vi "Configure Limit Test.vi"(0 "VISA resource name":refnum<visa-resource-name>, 1 "Upper Fail Line (0)":i32, 2 "Lower Fail Line (0)":i32, 5 "Limit Number (0: Limit1)":i32(ring) items=["Limit1", "Limit2"], 7 "Enable Limit Test (F: Disable)":bool, 9 "Upper Limit (1.000000E+0)":dbl=1.0 format="%.6e", 11 "error in (no error)":errorcluster, 12 "Lower Limit (-1.000000E+0)":dbl=-1.0 format="%.6e", 13 "Auto Clear (T: Enable)":bool=TRUE) -> (4 "VISA resource name out":refnum<visa-resource-name>, 15 "error out":errorcluster)   [LabVIEW 2016, in "Keithley 6517.lvlib"]
doc: "Configures the LIMIT 1 or 2 for CALC 3(model 6517) or CALC2(model 6514) math calculation."
uses:
  <instrlib>/Keithley 6517/Keithley 6517.lvlib
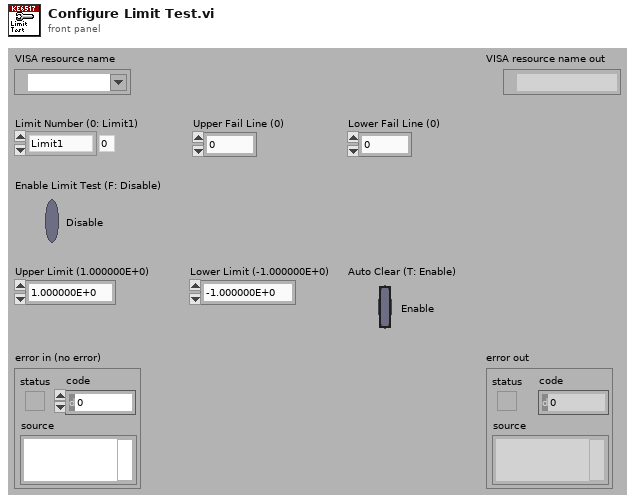
[diagram p1: front panel]
types:
  T1 = typedef "Keithley 6517.lvlib/Extended User Data.ctl" = cluster{"Instrument Model":i32}
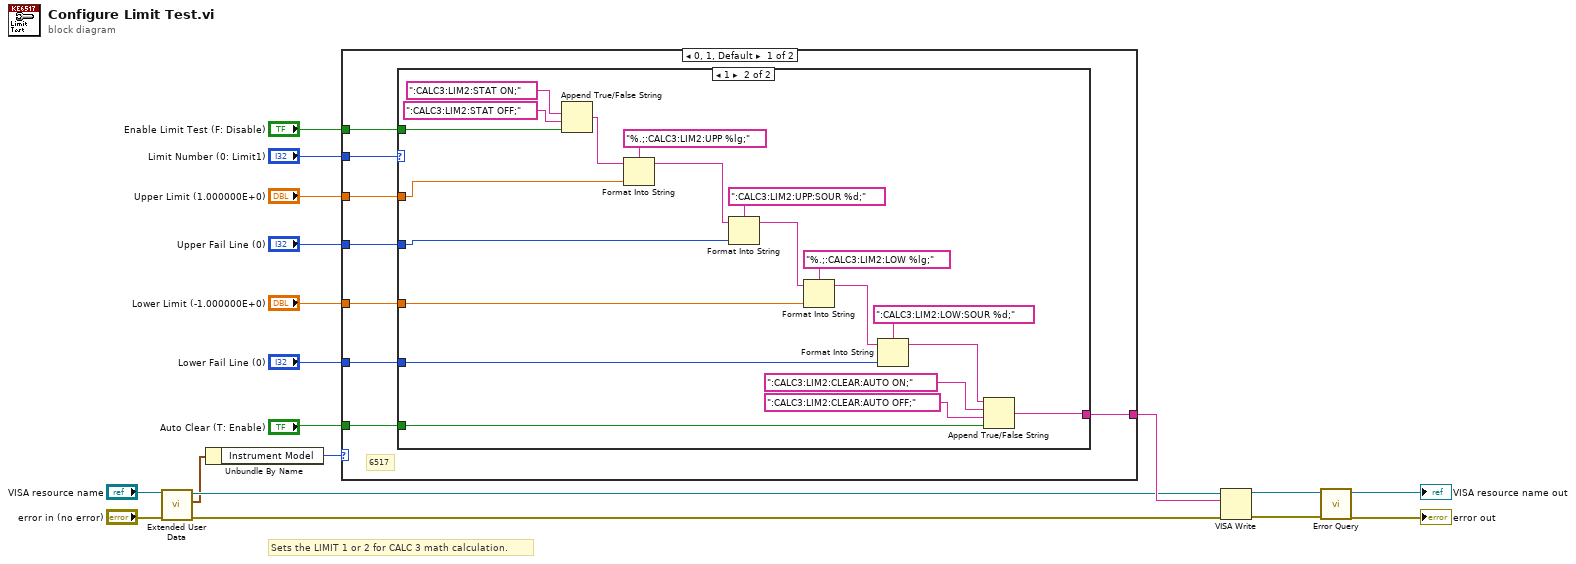
[diagram p0: block diagram]
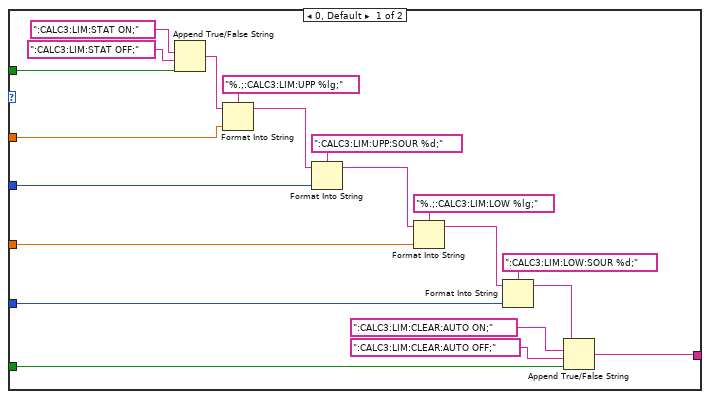
[diagram p2: hidden frame]
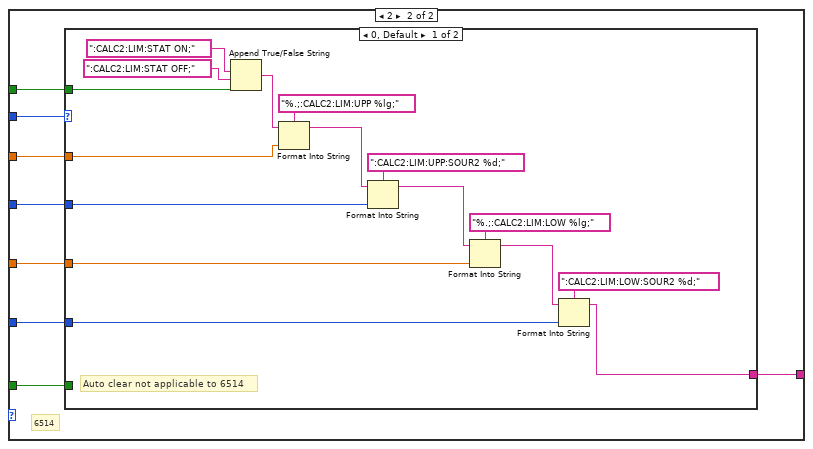
[diagram p3: hidden frame]
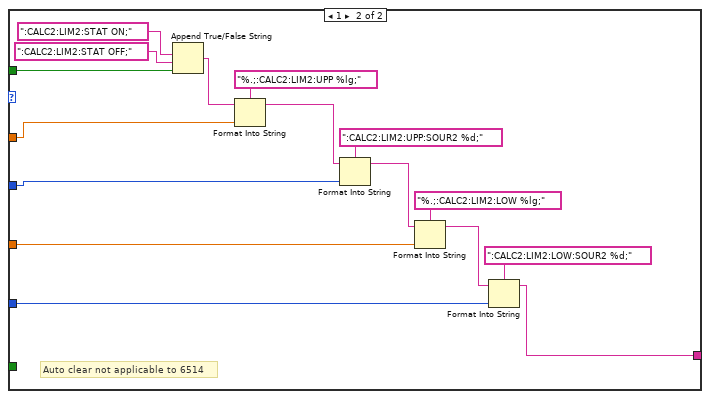
[diagram p4: hidden frame]
diagram:
  # "Sets the LIMIT 1 or 2 for CALC 3 math calculation."
  n1 = call <instrlib>:"Extended User Data.vi"("error in (no error)"="error in (no error)", "VISA resource name"="VISA resource name") -> ("error out"=w4:errorcluster, "User Data Out"=w2:T1, "VISA resource name out"=w3:refnum<visa-resource-name>)  [unwired: 7 in]
  n2 = Unbundle By Name(w2) -> ("Instrument Model"=w1:i32)
  n3 = case shown="0, 1, Default" w1 {
    tunnel: "Enable Limit Test (F: Disable)" -> [w26 w74]
    tunnel: "Limit Number (0: Limit1)" -> [w25 w73]
    tunnel: "Upper Limit (1.000000E+0)" -> [w24 w72]
    tunnel: "Upper Fail Line (0)" -> [w23 w71]
    tunnel: "Lower Limit (-1.000000E+0)" -> [w22 w70]
    tunnel: "Lower Fail Line (0)" -> [w21 w69]
    tunnel: "Auto Clear (T: Enable)" -> [w20 w68]
    tunnel: [w19 w67] -> w7
    frame 0, 1, Default {
      # "6517"
      n4 = case shown="1" w25 {
        tunnel: w26 -> [w33 w53]
        tunnel: w24 -> [w32 w52]
        tunnel: w23 -> [w31 w50]
        tunnel: w22 -> [w30 w47]
        tunnel: w21 -> [w29 w48]
        tunnel: w20 -> [w28 w49]
        tunnel: [w27 w51] -> w19
        frame 0, Default {
          n5 = Append True/False String(1:w33, 2:":CALC3:LIM:STAT OFF;", 3:":CALC3:LIM:STAT ON;") -> (0:w36:string)  [unwired: 1 in]
          n6 = Format Into String(format string="%.;:CALC3:LIM:UPP %lg;", initial string=w36, w32) -> (resulting string=w38:string)  [unwired: 1 in, 1 out]
          n7 = Format Into String(format string=":CALC3:LIM:UPP:SOUR %d;", initial string=w38, w31) -> (resulting string=w40:string)  [unwired: 1 in, 1 out]
          n8 = Format Into String(format string="%.;:CALC3:LIM:LOW %lg;", initial string=w40, w30) -> (resulting string=w42:string)  [unwired: 1 in, 1 out]
          n9 = Format Into String(format string=":CALC3:LIM:LOW:SOUR %d;", initial string=w42, w29) -> (resulting string=w44:string)  [unwired: 1 in, 1 out]
          n10 = Append True/False String(1:w28, 2:":CALC3:LIM:CLEAR:AUTO OFF;", 3:":CALC3:LIM:CLEAR:AUTO ON;", 4:w44) -> (0:w27:string)
        }
        frame 1 {
          n11 = Append True/False String(1:w53, 2:":CALC3:LIM2:STAT OFF;", 3:":CALC3:LIM2:STAT ON;") -> (0:w57:string)  [unwired: 1 in]
          n12 = Format Into String(format string="%.;:CALC3:LIM2:UPP %lg;", initial string=w57, w52) -> (resulting string=w58:string)  [unwired: 1 in, 1 out]
          n13 = Format Into String(format string=":CALC3:LIM2:UPP:SOUR %d;", initial string=w58, w50) -> (resulting string=w61:string)  [unwired: 1 in, 1 out]
          n14 = Format Into String(format string="%.;:CALC3:LIM2:LOW %lg;", initial string=w61, w47) -> (resulting string=w63:string)  [unwired: 1 in, 1 out]
          n15 = Format Into String(format string=":CALC3:LIM2:LOW:SOUR %d;", initial string=w63, w48) -> (resulting string=w64:string)  [unwired: 1 in, 1 out]
          n16 = Append True/False String(1:w49, 2:":CALC3:LIM2:CLEAR:AUTO OFF;", 3:":CALC3:LIM2:CLEAR:AUTO ON;", 4:w64) -> (0:w51:string)
        }
      }
    }
    frame 2 {
      # "6514"
      n17 = case shown="0, Default" w73 {
        tunnel: w74 -> [w80 w96]
        tunnel: w72 -> [w79 w95]
        tunnel: w71 -> [w78 w94]
        tunnel: w70 -> [w77 w92]
        tunnel: w69 -> [w76 w93]
        tunnel: w68 -> [_ _]
        tunnel: [w75 w91] -> w67
        frame 0, Default {
          # "Auto clear not applicable to 6514"
          n18 = Append True/False String(1:w80, 2:":CALC2:LIM:STAT OFF;", 3:":CALC2:LIM:STAT ON;") -> (0:w83:string)  [unwired: 1 in]
          n19 = Format Into String(format string="%.;:CALC2:LIM:UPP %lg;", initial string=w83, w79) -> (resulting string=w85:string)  [unwired: 1 in, 1 out]
          n20 = Format Into String(format string=":CALC2:LIM:UPP:SOUR2 %d;", initial string=w85, w78) -> (resulting string=w87:string)  [unwired: 1 in, 1 out]
          n21 = Format Into String(format string="%.;:CALC2:LIM:LOW %lg;", initial string=w87, w77) -> (resulting string=w89:string)  [unwired: 1 in, 1 out]
          n22 = Format Into String(format string=":CALC2:LIM:LOW:SOUR2 %d;", initial string=w89, w76) -> (resulting string=w75:string)  [unwired: 1 in, 1 out]
        }
        frame 1 {
          # "Auto clear not applicable to 6514"
          n23 = Append True/False String(1:w96, 2:":CALC2:LIM2:STAT OFF;", 3:":CALC2:LIM2:STAT ON;") -> (0:w100:string)  [unwired: 1 in]
          n24 = Format Into String(format string="%.;:CALC2:LIM2:UPP %lg;", initial string=w100, w95) -> (resulting string=w101:string)  [unwired: 1 in, 1 out]
          n25 = Format Into String(format string=":CALC2:LIM2:UPP:SOUR2 %d;", initial string=w101, w94) -> (resulting string=w104:string)  [unwired: 1 in, 1 out]
          n26 = Format Into String(format string="%.;:CALC2:LIM2:LOW %lg;", initial string=w104, w92) -> (resulting string=w106:string)  [unwired: 1 in, 1 out]
          n27 = Format Into String(format string=":CALC2:LIM2:LOW:SOUR2 %d;", initial string=w106, w93) -> (resulting string=w91:string)  [unwired: 1 in, 1 out]
        }
      }
    }
  }
  n28 = VISA Write(VISA resource name=w3, write buffer=w7, error in (no error)=w4) -> (VISA resource name out=w18:refnum<visa-resource-name>, error out=w17:errorcluster)  [unwired: 1 out]
  n29 = call <instrlib>:"Error Query.vi"("error in (no error)"=w17, "VISA resource name"=w18) -> ("error out"=→"error out":errorcluster, "VISA resource name out"=→"VISA resource name out":refnum<visa-resource-name>)  [unwired: 6 in, 2 out]
